vi "Gui_Set_Lists_Refs.vi"(8 "error in (no error)":errorcluster, 9 "Path":path, 10 "EXPERIMENT Inputs":T1={"Setup"="", "Date"="", "User Name"="", "Comment"="", "Experiment Procedures"=[], "Chemical Source"="", "Sample Components"=[], "Species"=[], "Laser 1"={"Used"=TRUE, "Name"="Spectroscopy", "Wavelength"=1000.0, "Energy"=25.0}, "Laser 2"={"Used"=TRUE, "Name"="Spectroscopy", "Wavelength"=1000.0, "Energy"=25.0}, "Laser 3"={"Used"=TRUE, "Name"="Spectroscopy", "Wavelength"=1000.0, "Energy"=25.0}, "Laser 4"={"Used"=TRUE, "Name"="Spectroscopy", "Wavelength"=1000.0, "Energy"=25.0}, "Laser 5"={"Used"=TRUE, "Name"="Spectroscopy", "Wavelength"=1000.0, "Energy"=25.0}, "Lamp 1"={"Used"=TRUE, "Name"="Spectroscopy", "Wavelength"=1000.0, "Attenuation"=25.0}, "Lamp 2"={"Used"=TRUE, "Name"="Spectroscopy", "Wavelength"=1000.0, "Attenuation"=25.0}, "Gas 1"={"Used"=TRUE, "Name"="Spectroscopy", "Pressure"=1000.0}, "Gas 2"={"Used"=TRUE, "Name"="Spectroscopy", "Pressure"=1000.0}, "Gas 3"={"Used"=TRUE, "Name"="Spectroscopy", "Pressure"=1000.0}, "Gas 4"={"Used"=TRUE, "Name"="Spectroscopy", "Pressure"=1000.0}, "Gas 5"={"Used"=TRUE, "Name"="Spectroscopy", "Pressure"=1000.0}}, 11 "Lists Refs":refnum<vi>[](array[refnum])) -> (0 "error out":errorcluster caption="sortie d'erreur", 3 "Lists Refs out":refnum<vi>[](array[refnum]))   [LabVIEW 2017]
uses:
  controls/EXPERIMENT_Inputs.ctl
  controls/LASER_Inputs.ctl
  controls/LAMP_Inputs.ctl
  controls/GAS_Inputs.ctl
panel:
  in  "Ref stricte":refnum<vi>
  # "Lasers"
  # "nm"
  # "mJ"
  # "Lamps"
  # "nm"
  # "dB"
  # "Gas"
  # "bar"
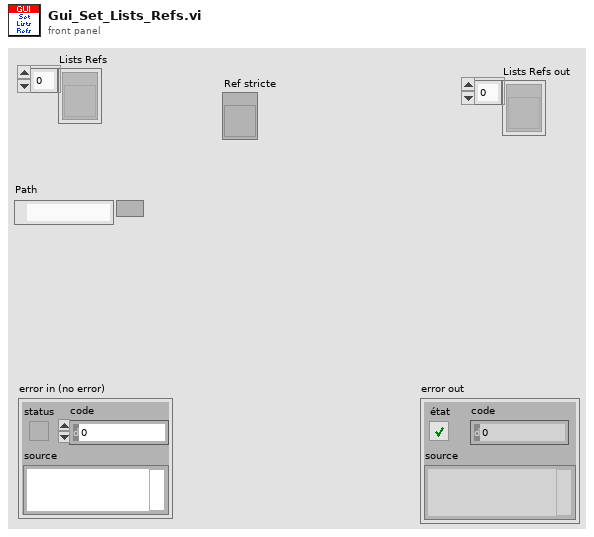
[diagram p1: front panel]
types:
  T1 = typedef "EXPERIMENT_Inputs.ctl" = cluster{"Setup":string, "Date":string, "User Name":string, "Comment":string, "Experiment Procedures":string[], "Chemical Source":string, "Sample Components":string[], "Species":string[], "Laser 1":T2, "Laser 2":T2, "Laser 3":T2, "Laser 4":T2, "Laser 5":T2, "Lamp 1":T3, "Lamp 2":T3, "Gas 1":T4, "Gas 2":T4, "Gas 3":T4, "Gas 4":T4, "Gas 5":T4}
  T2 = typedef "LASER_Inputs.ctl" = cluster{"Used":bool, "Name":string, "Wavelength":dbl, "Energy":dbl}
  T3 = typedef "LAMP_Inputs.ctl" = cluster{"Used":bool, "Name":string, "Wavelength":dbl, "Attenuation":dbl}
  T4 = typedef "GAS_Inputs.ctl" = cluster{"Used":bool, "Name":string, "Pressure":dbl}
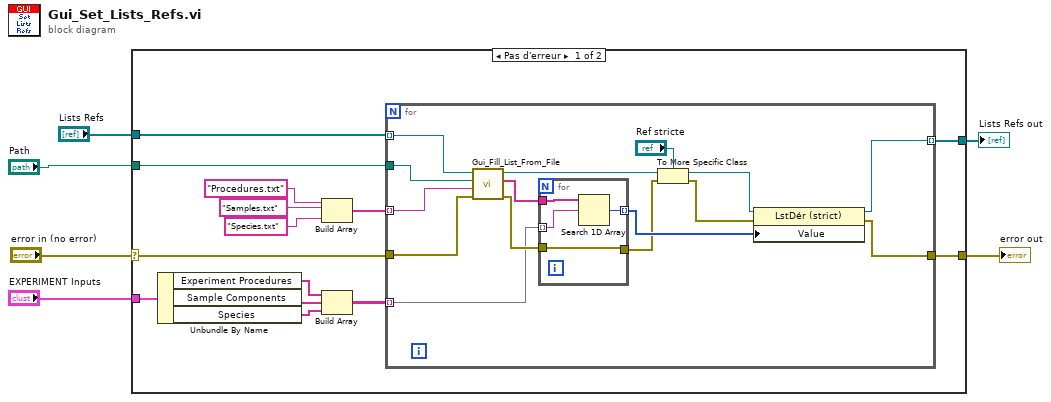
[diagram p0: block diagram]
diagram:
  n1 = case shown="Pas d'erreur" "error in (no error)" {
    selector: "error in (no error)" -> [w20 w41]
    tunnel: [w7 w41] -> w6
    tunnel: "Lists Refs" -> [w15 w40]
    tunnel: [w8 w40] -> w1
    tunnel: "Path" -> [w14 _]
    tunnel: "EXPERIMENT Inputs" -> [w13 _]
    frame No Error {
      n2 = Unbundle By Name(w13) -> ("Experiment Procedures"=w17:string[], "Sample Components"=w18:string[], "Species"=w19:string[])
      n3 = Build Array("Procedures.txt", "Samples.txt", "Species.txt") -> (w9:string[])
      n4 = Build Array(w17, w18, w19) -> (w16:string[][])
      n5 = for {
        tunnel: w16 -> [w29] mode=indexing
        tunnel: w15 -> [w33] mode=indexing
        tunnel: w20 -> [w32]
        tunnel: w14 -> [w35]
        tunnel: w9 -> [w34] mode=indexing
        tunnel: [w27] -> w8 mode=indexing
        tunnel: [w21] -> w7
        n6 = call "Gui_Fill_List_From_File.vi"("error in (no error)"=w32, "Resource Name"=w34, "Resource Path"=w35, "Refnum LstDér"=w33) -> ("error out"=w31:errorcluster, "Table"=w30:string[], "Refnum LstDér out"=w25:refnum<vi>)  [unwired: 5 in]
        n7 = for {
          tunnel: w30 -> [w37]
          tunnel: [w39] -> w28 mode=indexing
          tunnel: w31 -> [w38]
          tunnel: [w38] -> w23
          tunnel: w29 -> [w36] mode=indexing
          n8 = Search 1D Array(1D array=w37, element=w36) -> (index of element=w39:i32)  [unwired: 1 in]
        }
        n9 = To More Specific Class(target class="Ref stricte", reference=w25, error in=w23) -> (specific class reference=w24:refnum<vi>, error out=w22:errorcluster)
        n10 = property on="Nœud de propriété" class="LstDér (strict)"(reference=w24, error in=w22, "Value"=w28) -> (reference out=w27:refnum<vi>, error out=w21:errorcluster)
      }
    }
    frame Error {
    }
  }
  "error out" <- w6
  "Lists Refs out" <- w1
